vi "Configure Trigger (Serial).vi"(0 "VISA resource name":refnum<visa-resource-name>, 1 "Clock Level (0.0V)":dbl, 2 "Clock Polarity(0:Positive)":u16(ring) items=["Positive", "Negative"], 3 "Standard (0:GB Ethernet)":u16(ring) items=["GB Ethernet", "FC133", "FC266", "FC531", "FC1063", "OC1", "OC3", "OC12", "FW1394BS400B", "FW1394BS800B", "ENET100FX", "RIO_500M", "RIO_750M", "RIO_1G", "RIO_SERIAL_1G", "VSROC192", "Custom"], 5 "Data Source":T1 {"Data Source (0:Channel1)" items=["Channel1", "Channel2", "Channel3", "Channel4"]}, 7 "Clock Source (14:Recovered Clock)":u16(ring)=14 items=["Channel1"=0, "Channel2"=1, "Channel3"=2, "Channel4"=3, "Recovered Clock"=14], 9 "Coding (0:NRZ)":u16(ring) items=["NRZ", "S8B10B"], 11 "error in (no error)":errorcluster, 12 "Bit Rate (155.5Mb/s)":dbl=155000000.0, 13 "Data Value  (XXXXXXXXXXXXXXXXXXXXXXXXXXXXXX01)":string="XXXXXXXXXXXXXXXXXXXXXXXXXXXXXX01" caption="Data Value") -> (4 "VISA resource name out":refnum<visa-resource-name>, 15 "error out":errorcluster)   [LabVIEW 2012, in "Tektronix 7000 Series.lvlib"]
doc: "Configures Serial trigger settings for an oscilloscope. A Serial trigger occurs when NRZ-encoded data up to 1.25 Gbaud is found, providing a 32¨Cbit serial word.\n\nTDS5000 and TDS5000B series oscilloscopes don't support Serial Trigger."
uses:
  Tektronix 7000 Series.lvlib
panel:
  # "msb"
  # "lsb"
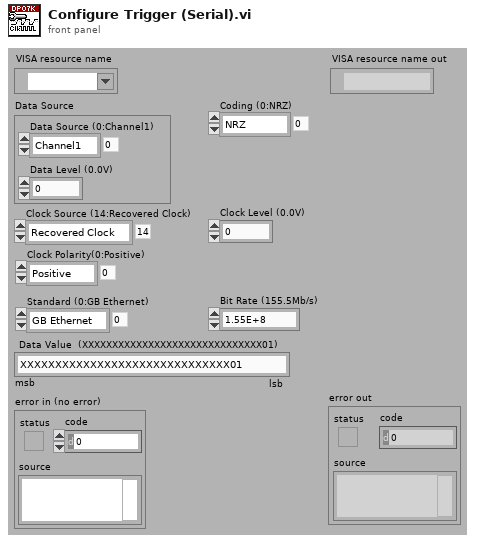
[diagram p1: front panel]
types:
  T1 = cluster{"Data Source (0:Channel1)":u16, "Data Level (0.0V)":dbl}
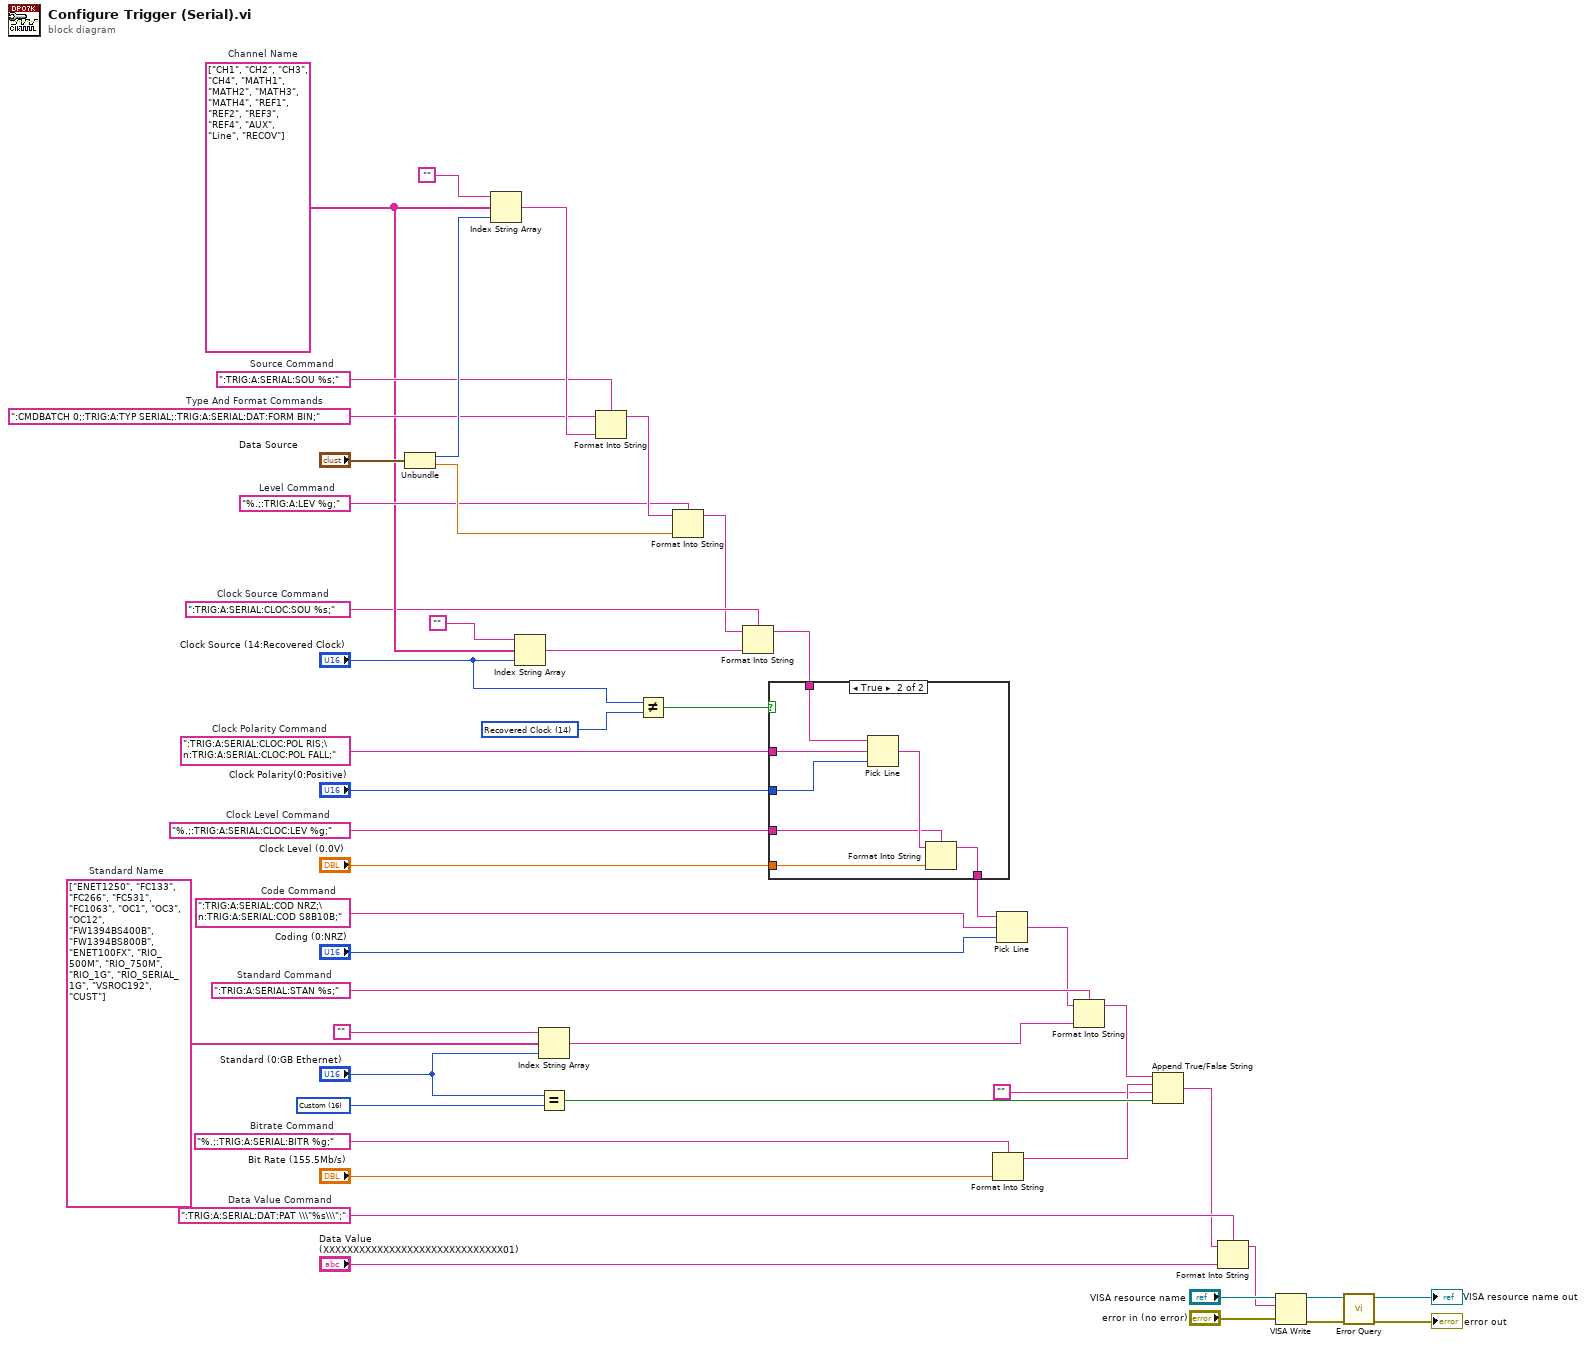
[diagram p0: block diagram]
diagram:
  w11 = "%.;:TRIG:A:SERIAL:BITR %g;"  # Bitrate Command
  w15 = u16 16 items=["GB Ethernet", "FC133", "FC266", "FC531", "FC1063", "OC1", "OC3", "OC12", "FW1394BS400B", "FW1394BS800B", "ENET100FX", "RIO_500M", "RIO_750M", "RIO_1G", "RIO_SERIAL_1G", "VSROC192", "Custom"] ("Standard (0:GB Ethernet)")
  w18 = ":TRIG:A:SERIAL:STAN %s;"  # Standard Command
  w21 = string[] ["ENET1250", "FC133", "FC266", "FC531", "FC1063", "OC1", "OC3", "OC12", "FW1394BS400B", "FW1394BS800B", "ENET100FX", "RIO_500M", "RIO_750M", "RIO_1G", "RIO_SERIAL_1G", "VSROC192", "CUST"]  # Standard Name
  w22 = ":TRIG:A:SERIAL:DAT:PAT \\\"%s\\\";"  # Data Value Command
  w25 = ":TRIG:A:SERIAL:COD NRZ;\n:TRIG:A:SERIAL:COD S8B10B;"  # Code Command
  w28 = "%.;:TRIG:A:SERIAL:CLOC:LEV %g;"  # Clock Level Command
  w34 = ":TRIG:A:SERIAL:CLOC:POL RIS;\n:TRIG:A:SERIAL:CLOC:POL FALL;"  # Clock Polarity Command
  w29 = u16 14 items=["Channel1"=0, "Channel2"=1, "Channel3"=2, "Channel4"=3, "Recovered Clock"=14] ("Clock Source (14:Recovered Clock)")
  w36 = ":TRIG:A:SERIAL:CLOC:SOU %s;"  # Clock Source Command
  w40 = "%.;:TRIG:A:LEV %g;"  # Level Command
  w43 = ":TRIG:A:SERIAL:SOU %s;"  # Source Command
  w44 = ":CMDBATCH 0;:TRIG:A:TYP SERIAL;:TRIG:A:SERIAL:DAT:FORM BIN;"  # Type And Format Commands
  w39 = string[] ["CH1", "CH2", "CH3", "CH4", "MATH1", "MATH2", "MATH3", "MATH4", "REF1", "REF2", "REF3", "REF4", "AUX", "Line", "RECOV"]  # Channel Name
  n1 = Unbundle("Data Source") -> ("Data Source (0:Channel1)"=w47:u16, "Data Level (0.0V)"=w41:dbl)
  n2 = Index String Array(1:w47, 2:w39, 3:"") -> (0:w45:string)
  n3 = Index String Array(1:"Clock Source (14:Recovered Clock)", 2:w39, 3:"") -> (0:w37:string)
  n4 = Index String Array(1:"Standard (0:GB Ethernet)", 2:w21, 3:"") -> (0:w19:string)
  n5 = Equal?(x="Standard (0:GB Ethernet)", y=w15) -> (x = y?=w14:bool)
  n6 = Format Into String(format string=w43, initial string=w44, w45) -> (resulting string=w42:string)  [unwired: 1 in, 1 out]
  n7 = Not Equal?(x="Clock Source (14:Recovered Clock)", y=w29) -> (x != y?=w31:bool)
  n8 = Format Into String(format string=w40, initial string=w42, w41) -> (resulting string=w35:string)  [unwired: 1 in, 1 out]
  n9 = Format Into String(format string=w36, initial string=w35, w37) -> (resulting string=w32:string)  [unwired: 1 in, 1 out]
  n10 = case shown="True" w31 {
    tunnel: w34 -> [_ w56]
    tunnel: "Clock Polarity(0:Positive)" -> [_ w55]
    tunnel: w32 -> [w49 w54]
    tunnel: w28 -> [_ w52]
    tunnel: "Clock Level (0.0V)" -> [_ w51]
    tunnel: [w49 w50] -> w26
    frame False {
    }
    frame True {
      n11 = Pick Line(string ("")=w54, multi-line string=w56, line index=w55) -> (output string=w53:string)
      n12 = Format Into String(format string=w52, initial string=w53, w51) -> (resulting string=w50:string)  [unwired: 1 in, 1 out]
    }
  }
  n13 = Format Into String(format string=w11, "Bit Rate (155.5Mb/s)") -> (resulting string=w10:string)  [unwired: 2 in, 1 out]
  n14 = Pick Line(string ("")=w26, multi-line string=w25, line index="Coding (0:NRZ)") -> (output string=w17:string)
  n15 = Format Into String(format string=w18, initial string=w17, w19) -> (resulting string=w13:string)  [unwired: 1 in, 1 out]
  n16 = Append True/False String(1:w14, 2:"", 3:w10, 4:w13) -> (0:w2:string)
  n17 = Format Into String(format string=w22, initial string=w2, "Data Value  (XXXXXXXXXXXXXXXXXXXXXXXXXXXXXX01)") -> (resulting string=w1:string)  [unwired: 1 in, 1 out]
  n18 = VISA Write(VISA resource name="VISA resource name", write buffer=w1, error in (no error)="error in (no error)") -> (VISA resource name out=w8:refnum<visa-resource-name>, error out=w7:errorcluster)  [unwired: 1 out]
  n19 = call "Error Query.vi"("error in (no error)"=w7, "VISA resource name"=w8) -> ("error out"=→"error out":errorcluster, "VISA resource name out"=→"VISA resource name out":refnum<visa-resource-name>)  [unwired: 6 in, 2 out]
